vi "Cal File Write System Cal Data Sections.vi"(6 "DATA":dbl[][](array[numeric]), 7 "DATA SECTION":T2, 8 "error in (no error)":errorcluster, 11 "Cal Ref":T1) -> (0 "error out":errorcluster, 3 "Cal Ref out":T1)   [LabVIEW 2011]
uses:
  <vilib>/Utility/config.llb/Config Data RefNum.ctl
  Module Cal File Section.ctl
  <vilib>/Utility/config.llb/Write Key (String).vi
  <vilib>/Utility/config.llb/NI_LVConfig.lvlib
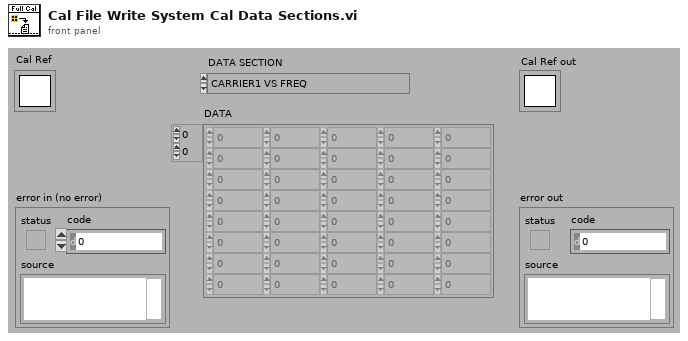
[diagram p1: front panel]
types:
  T1 = typedef "NI_LVConfig.lvlib/Config Data RefNum.ctl" = refnum<k1>
  T2 = typedef "Module Cal File Section.ctl" = enum16{"CARRIER1 VS FREQ", "CARRIER2 VS FREQ", "PAD1 VS FREQUENCY", "PAD2 VS FREQUENCY", "RX POWER VS FREQUENCY", "PORT 3 VS ATTENUATION", "PORT 3 VS FREQUENCY", "HIGH POWER PAD VS FREQUENCY", "D1 VS ATTENUATION", "D1 VS FREQUENCY", "D2 VS ATTENUATION", "D2 VS FREQUENCY", "D1 LOSS VS FREQUENCY", "D2 LOSS VS FREQUENCY", "RX REVERSE", "RX FORWARD", "RX AUXILIARY", "TXA", "TXB", "TXC", "RXA", "RXB", "RXC", "RXD", "RXE", "RXF"}
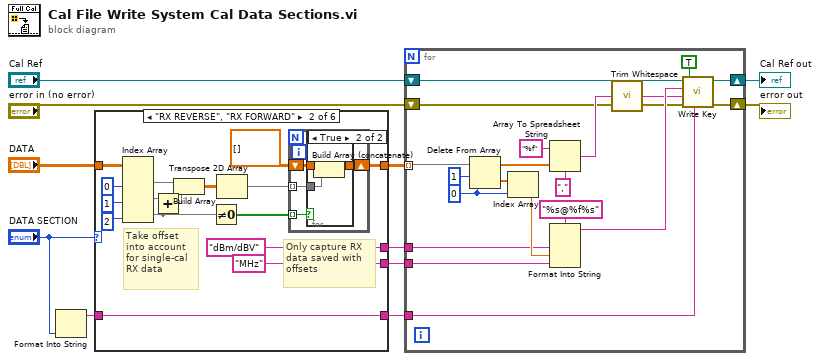
[diagram p0: block diagram]
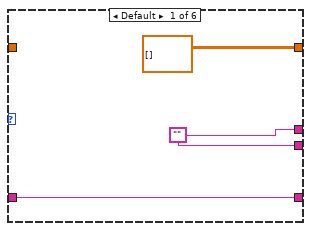
[diagram p2: hidden frame]
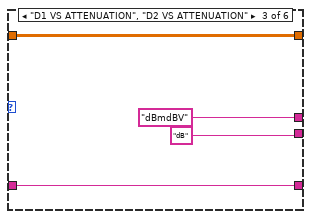
[diagram p4: hidden frame]
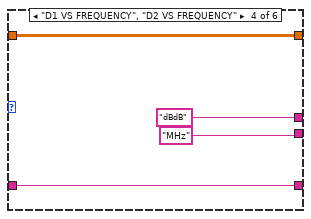
[diagram p5: hidden frame]
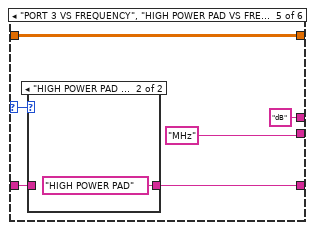
[diagram p6: hidden frame]
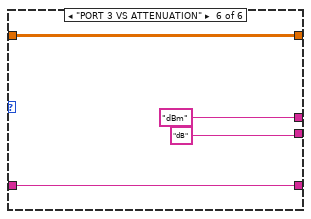
[diagram p8: hidden frame]
diagram:
  n1 = Format Into String("DATA SECTION") -> (resulting string=w1:string)  [unwired: 3 in, 1 out]
  n2 = case shown="\"RX REVERSE\", \"RX FORWARD\"" "DATA SECTION" {
    selector: "DATA SECTION" -> [_ _ _ _ w49 _]
    tunnel: [w13 "dBm/dBV" ("Key Name Prefix") "dBmdBV" ("Key Name Prefix") "dBdB" ("Key Name Prefix") "dB" ("Key Name Prefix") "dBm" ("Key Name Prefix")] -> w11
    tunnel: [w13 "MHz" ("Key Name Suffix") "dB" ("Key Name Suffix") "MHz" ("Key Name Suffix") "MHz" ("Key Name Suffix") "dB" ("Key Name Suffix")] -> w10
    tunnel: "DATA" -> [_ w27 w40 w44 w50 w56]
    tunnel: [dbl[][] [] ("DATA") w15 w40 w44 w50 w56] -> w5
    tunnel: [w12 w28 w39 w43 w48 w55] -> w3
    tunnel: w1 -> [w12 w28 w39 w43 w47 w55]
    frame Default {
      w13 = ""
    }
    frame "RX REVERSE", "RX FORWARD" {
      # "Take offset into account for single-cal RX data"
      # "Only capture RX data saved with \noffsets"
      n3 = Index Array(array=w27, index (col) #1=0 ("disabled index (col)"), index (col) #2=1 ("disabled index (col)"), index (col) #3=2 ("disabled index (col)")) -> (element #1=w22:dbl[], element #2=w23:dbl[], element #3=w19:dbl[])  [unwired: 3 in]
      n4 = Add(x=w23, y=w19) -> (x+y=w20:dbl[])
      n5 = Build Array(w22, w20) -> (w21:dbl[][])
      n6 = Not Equal To 0?(x=w19) -> (x != 0?=w16:bool[])
      n7 = Transpose 2D Array(2D array=w21) -> (transposed array=w17:dbl[][])
      n8 = for {
        shift-right: [w31] -> w15
        shift-left: dbl[][] [] ("DATA") -> [w32]
        tunnel: w17 -> [w33] mode=indexing
        tunnel: w16 -> [w34] mode=indexing
        n9 = case shown="True" w34 {
          tunnel: w33 -> [_ w37]
          tunnel: w32 -> [w35 w38]
          tunnel: [w35 w36] -> w31
          frame False {
          }
          frame True {
            n10 = Build Array (concatenate)(w38, w37) -> (w36:dbl[][])
          }
        }
      }
    }
    frame "D1 VS ATTENUATION", "D2 VS ATTENUATION" {
    }
    frame "D1 VS FREQUENCY", "D2 VS FREQUENCY" {
    }
    frame "PORT 3 VS FREQUENCY", "HIGH POWER PAD VS FREQUENCY" {
      n11 = case shown="\"HIGH POWER PAD VS FREQUENCY\"" w49 {
        tunnel: [w53 "HIGH POWER PAD" ("Key Name Suffix")] -> w48
        tunnel: w47 -> [w53 _]
        frame Default {
        }
        frame "HIGH POWER PAD VS FREQUENCY" {
        }
      }
    }
    frame "PORT 3 VS ATTENUATION" {
    }
  }
  n12 = for {
    tunnel: w5 -> [w78] mode=indexing
    tunnel: w11 -> [w69]
    tunnel: w10 -> [w68]
    shift-right: [w63] -> w7
    shift-left: "error in (no error)" -> [w64]
    shift-right: [w62] -> w4
    shift-left: "Cal Ref" -> [w67]
    tunnel: w3 -> [w61]
    w75 = 0 ("index")
    n13 = Delete From Array(array=w78, length=1, index=w75) -> (deleted portion=w76:dbl[], array with subset deleted=w72:dbl[])
    n14 = Index Array(array=w76, index=w75) -> (element=w70:dbl)
    n15 = Array To Spreadsheet String(delimiter (Tab)=",", array=w72, 3:"%f" ("format string")) -> (spreadsheet string=w65:string)
    n16 = Format Into String(format string="%s@%f%s", w69, w70, w68) -> (resulting string=w66:string)  [unwired: 2 in, 1 out]
    n17 = call <vilib>:"Trim Whitespace.vi"("string"=w65) -> ("trimmed string"=w60:string)  [unwired: 1 in]
    n18 = call-poly <vilib>:"Write Key.vi"("write raw string? (F)"=TRUE, "section"=w61, "error in (no error)"=w64, "value"=w60, "key"=w66, "refnum"=w67) -> ("error out"=w63:errorcluster, "refnum out"=w62:T1)  [unwired: 3 in, 1 out]
  }
  "error out" <- w7
  "Cal Ref out" <- w4
